vi "tidyNamespaceAttribute.vi"(8 "error in (no error)":errorcluster, 10 "Fully Qualified String":string="TCS.lvlib:TCSDataDefinitions.lvlib:TCSCommand.lvlib:AzElTarget.lvclass", 11 "AttributeWriter In":refnum<class "XMLAttributeGenerator.lvclass">) -> (0 "error out":errorcluster, 2 "attributeData":T1, 3 "AttributeWriter Out":refnum<class "XMLAttributeGenerator.lvclass">)   [LabVIEW 2016, in "XML.lvlib" / "XMLAttributeGenerator.lvclass"]
doc: "This method cleans up the LabVIEW namespace by removing any file extensions like .lvlib and .lvclass for example."
uses:
  <userlib>/Common/XML/XMLAttributeGenerator/XMLAttributeGenerator.lvclass
  <userlib>/Common/XML/Typedefs/AttributeElements.ctl
  <userlib>/Common/XML/XML.lvlib
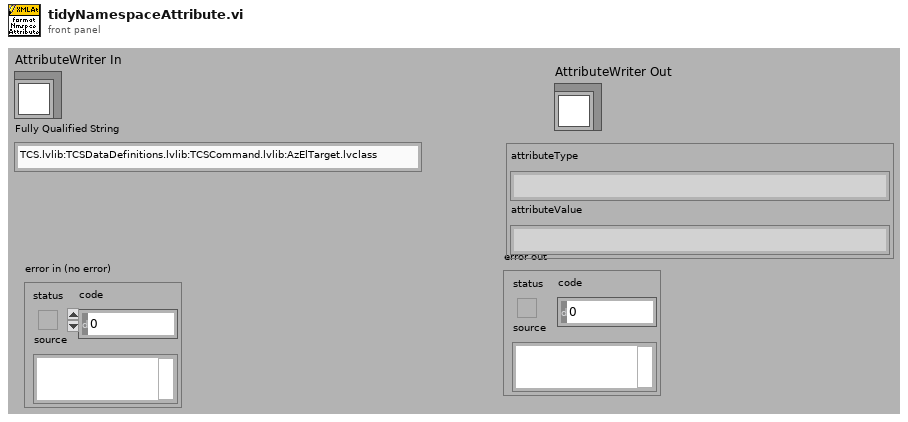
[diagram p1: front panel]
types:
  T1 = typedef "XML.lvlib/AttributeElements.ctl" = cluster{"attributeType":string, "attributeValue":string}
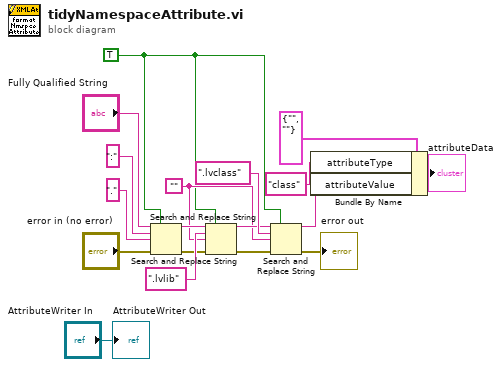
[diagram p0: block diagram]
diagram:
  w12 = ""
  w4 = TRUE ("replace all? (F)")
  n1 = Search and Replace String(replace all?=w4, input string="Fully Qualified String", search string=":", replace string="." ("replace string (\"\")"), error in="error in (no error)") -> (result string=w16:string, error out=w10:errorcluster)  [unwired: 3 in, 2 out]
  n2 = Search and Replace String(replace all?=w4, input string=w16, search string=".lvlib", replace string=w12, error in=w10) -> (result string=w13:string, error out=w9:errorcluster)  [unwired: 3 in, 2 out]
  n3 = Search and Replace String(replace all?=w4, input string=w13, search string=".lvclass", replace string=w12, error in=w9) -> (result string=w3:string, error out=→"error out":errorcluster)  [unwired: 3 in, 2 out]
  n4 = Bundle By Name(cluster=T1 {"attributeType"="", "attributeValue"=""} ("attributeData 2"), "attributeType"="class", "attributeValue"=w3) -> (→"attributeData":T1)
  "AttributeWriter Out" <- "AttributeWriter In"
